vi "sub_ycar_serial-data-buff.vi"(7 "cmd":T1, 10 "serial buffer n":i32, 11 "data":string) -> (2 "data":string, 3 "val":bool)   [LabVIEW 2019]
uses:
  Ctrl/cmd_common.ctl
panel:
  in  "Led":bool
  out "send_data":u8[](array[numeric]) format="%x"
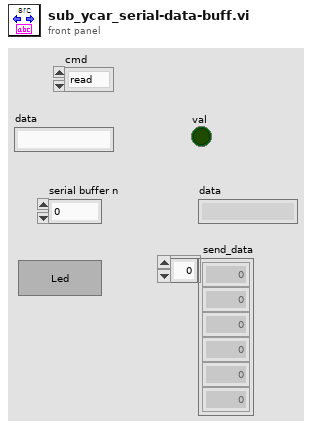
[diagram p1: front panel]
types:
  T1 = typedef "cmd_common.ctl" = enum16{"read", "write"}
  T2 = typedef "joystick_opval.ctl" = cluster{"curr":u32, "last":u32}
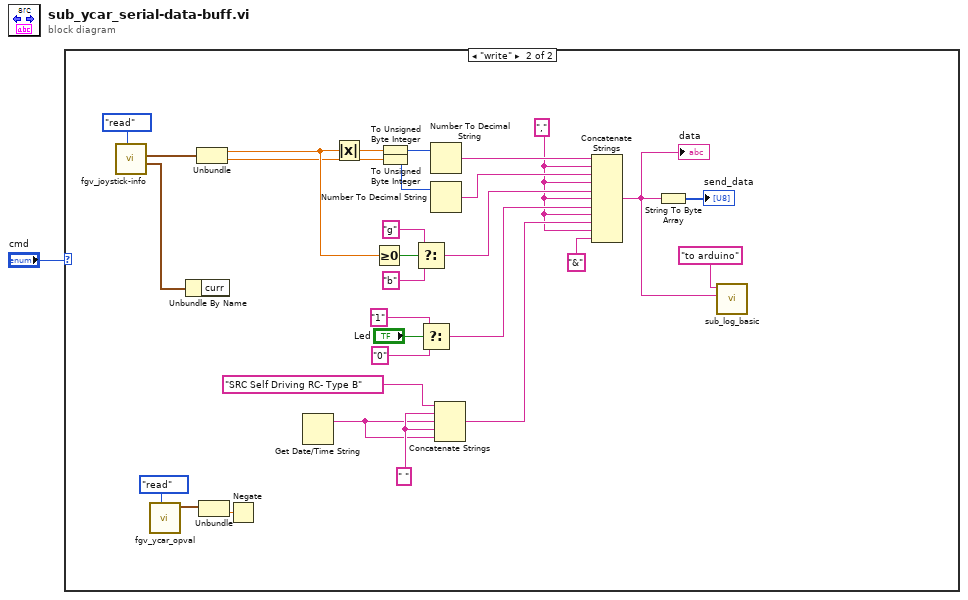
[diagram p0: block diagram]
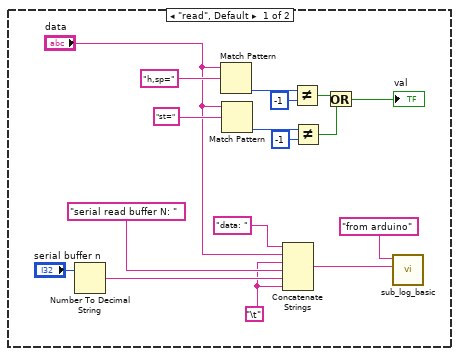
[diagram p2: hidden frame]
diagram:
  n1 = case shown="\"write\"" "cmd" {
    frame "read", Default {
      w5 = "\t"
      n2 = Number To Decimal String(number="serial buffer n") -> (decimal integer string=w7:string)  [unwired: 1 in]
      n3 = Match Pattern(string="data", regular expression="h,sp=") -> (offset past match=w17:i32)  [unwired: 1 in, 3 out]
      n4 = Match Pattern(string="data", regular expression="st=") -> (offset past match=w14:i32)  [unwired: 1 in, 3 out]
      n5 = Concatenate Strings("data: " ("문자열"), "data", w5, "serial read buffer N: " ("문자열"), w7, w5) -> (w4:string)
      n6 = Not Equal?(x=w17, y=-1) -> (x != y?=w12:bool)
      n7 = Not Equal?(x=w14, y=-1) -> (x != y?=w13:bool)
      n8 = Or(x=w12, y=w13) -> (x .or. y?=→"val":bool)
      n9 = call "sub_log_basic.vi"("desc"=w4, "Title"="from arduino") -> ()  [unwired: 9 in, 1 out]
    }
    frame "write" {
      w28 = " " ("문자열")
      w21 = "," ("string")
      n10 = call "fgv_joystick-info.vi"("init"=enum16{"enable", "init", "read", "write"}."read") -> ("opval"=w19:T2, "v_val"=w20:cluster{dbl, dbl})  [unwired: 7 in, 2 out]
      n11 = call "fgv_ycar_opval.vi"("cmd"=enum16{"read", "write", "ini"}."read") -> ("opval out"=w34:cluster{"speed":dbl, "steer":dbl})  [unwired: 10 in]
      n12 = Unbundle By Name(w19) -> ()  [unwired: 1 out]
      n13 = Unbundle(w20) -> (w37:dbl, w32:dbl)
      n14 = Unbundle(w34) -> ("steer"=w33:dbl)  [unwired: 1 out]
      n15 = Negate(x=w33) -> ()  [unwired: 1 out]
      n16 = Get Date/Time String() -> (date string=w27:string)  [unwired: 3 in, 1 out]
      n17 = Absolute Value(x=w37) -> (abs(x)=w36:dbl)
      n18 = Greater Or Equal To 0?(x=w37) -> (x >= 0?=w41:bool)
      n19 = To Unsigned Byte Integer(number=w36) -> (unsigned 8bit integer=w44:u8)
      n20 = To Unsigned Byte Integer(number=w32) -> (unsigned 8bit integer=w43:u8)
      n21 = Select(t="g" ("string"), s=w41, f="b" ("string")) -> (s? t:f=w38:string)
      n22 = Select(t="1" ("string"), s="Led", f="0" ("string")) -> (s? t:f=w22:string)
      n23 = Number To Decimal String(number=w44) -> (decimal integer string=w47:string)  [unwired: 1 in]
      n24 = Number To Decimal String(number=w43) -> (decimal integer string=w45:string)  [unwired: 1 in]
      n25 = Concatenate Strings("SRC Self Driving RC- Type B" ("문자열"), w28, w27, w28, w27) -> (w26:string)
      n26 = Concatenate Strings(w47, w21, w45, w21, w38, w21, w22, w21, w26, w21, "&" ("string")) -> (w30:string)
      "data" <- w30
      n27 = String To Byte Array(string=w30) -> (unsigned byte array=→"send_data":u8[])
      n28 = call "sub_log_basic.vi"("desc"=w30, "Title"="to arduino") -> ()  [unwired: 9 in, 1 out]
    }
  }
